vi "Write Datalog File.vi"(3 "points per acquisition":i32=100, 4 "number of acquisitions":i32=10, 5 "Data Log File Refnum":refnum<k1>) -> (0 "error out":errorcluster, 2 "Array Data Out":cluster{string, "empty array":sgl[]}[](array[cluster]) {"empty array" format="%0.2f"})   [LabVIEW 2012]
doc: "Creates a datalog file and writes a specified number of records to the datalog file. Each record is a cluster containing a timestamp string and an array of single-precision numbers."
panel:
  out "record data":sgl[](graph)
  out "record time":string
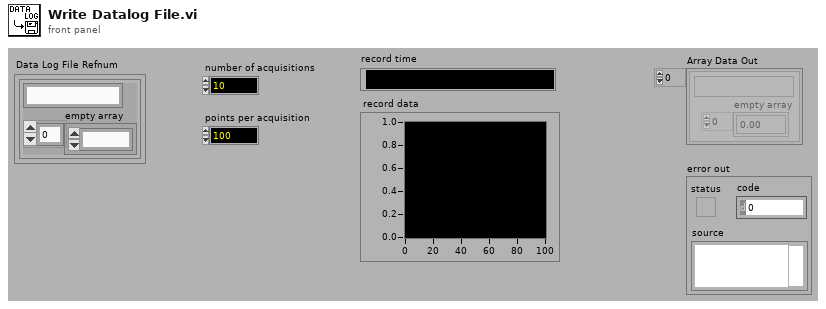
[diagram p1: front panel]
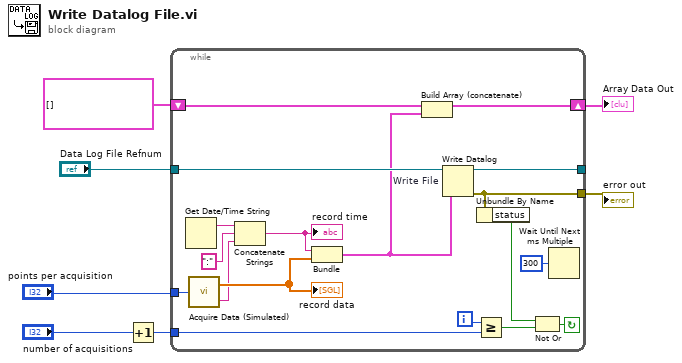
[diagram p0: block diagram]
diagram:
  n1 = Increment(x="number of acquisitions") -> (x+1=w6:i32)
  n2 = while {
    tunnel: [w15] -> _
    tunnel: "Data Log File Refnum" -> [w16]
    tunnel: [w22] -> w1
    tunnel: w6 -> [w17]
    tunnel: "points per acquisition" -> [w13]
    shift-right: [w8] -> w2
    shift-left: cluster{string, "empty array":sgl[]}[] [] -> [w10]
    i -> [w18]
    stop <- w19 continue-if-true
    n3 = Get Date/Time String() -> (date string=w23:string)  [unwired: 4 out]
    n4 = call "Acquire Data (Simulated).vi"("# of points"=w13) -> ("data"=w12:sgl[], "time"=w11:string)
    "record data" <- w12
    n5 = Concatenate Strings(w23, ":", w11) -> (w25:string)
    "record time" <- w25
    n6 = Bundle(w25, "data"=w12) -> (w9:cluster{string, "data":sgl[]})  [unwired: 1 out]
    n7 = Build Array (concatenate)(w10, w9) -> (w8:cluster{string, "data":sgl[]}[])
    n8 = Write Datalog "Write File"(6:w9, 7:w16) -> (0:w22:errorcluster, 3:w15:refnum<k1>)  [unwired: 1 in]
    n9 = Greater Or Equal?(x=w18, y=w17) -> (x >= y?=w20:bool)
    n10 = Unbundle By Name(w22) -> ("status"=w21:bool)
    n11 = Not Or(1:w20, 2:w21) -> (0:w19:bool)
    n12 = Wait Until Next ms Multiple(millisecond multiple=u32 300) -> ()  [unwired: 1 out]
  }
  "Array Data Out" <- w2
  "error out" <- w1
